vi "Status Display Configuration.vi"(0 "VISA resource name (in)":refnum<visa-resource-name>, 2 "Unit Address (-1)":i32=-1, 5 "error in (no error)":errorcluster, 6 "Retry Attempts (0)":i32 min=0) -> (14 "VISA resource name (out)":refnum<visa-resource-name>, 15 "Decimal Point":T4, 16 "Temperature Units":T3, 17 "Display Color":T2, 18 "Display Brightness":T1, 19 "error out":errorcluster)   [LabVIEW 2020, in "Omega Platinum Series.lvlib"]
doc: "Get the display configuration for the controller."
uses:
  <instrlib>/RxnRover/OmegaPlatinumSeriesDriver/Omega Platinum Series.lvlib
  <instrlib>/RxnRover/OmegaPlatinumSeriesDriver/Public/Type Defs/Display Decimal Point.ctl
  <instrlib>/RxnRover/OmegaPlatinumSeriesDriver/Public/Type Defs/Display Temperature Units.ctl
  <instrlib>/RxnRover/OmegaPlatinumSeriesDriver/Public/Type Defs/Display Color.ctl
  <instrlib>/RxnRover/OmegaPlatinumSeriesDriver/Public/Type Defs/Display Brightness.ctl
panel:
  out "Command":string
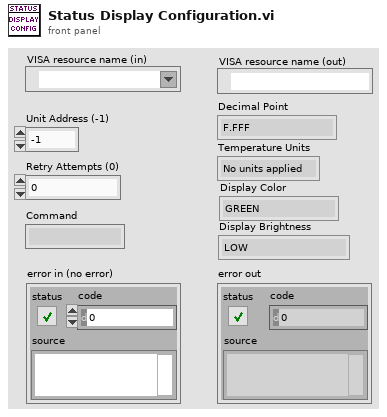
[diagram p1: front panel]
types:
  T1 = typedef "Omega Platinum Series.lvlib/Display Brightness.ctl" = enum16{"LOW", "MEDIUM", "HIGH"}
  T2 = typedef "Omega Platinum Series.lvlib/Display Color.ctl" = enum16{"GREEN", "RED", "AMBER"}
  T3 = typedef "Omega Platinum Series.lvlib/Display Temperature Units.ctl" = enum16{"No units applied", "Celsius", "Fahrenheit"}
  T4 = typedef "Omega Platinum Series.lvlib/Display Decimal Point.ctl" = enum16{"F.FFF", "FF.FF"}
  T5 = typedef "Omega Platinum Series.lvlib/Response.ctl" = cluster{"Unit Address":i32, "Command Class":string, "Command ID":u32, "Parameters":string}
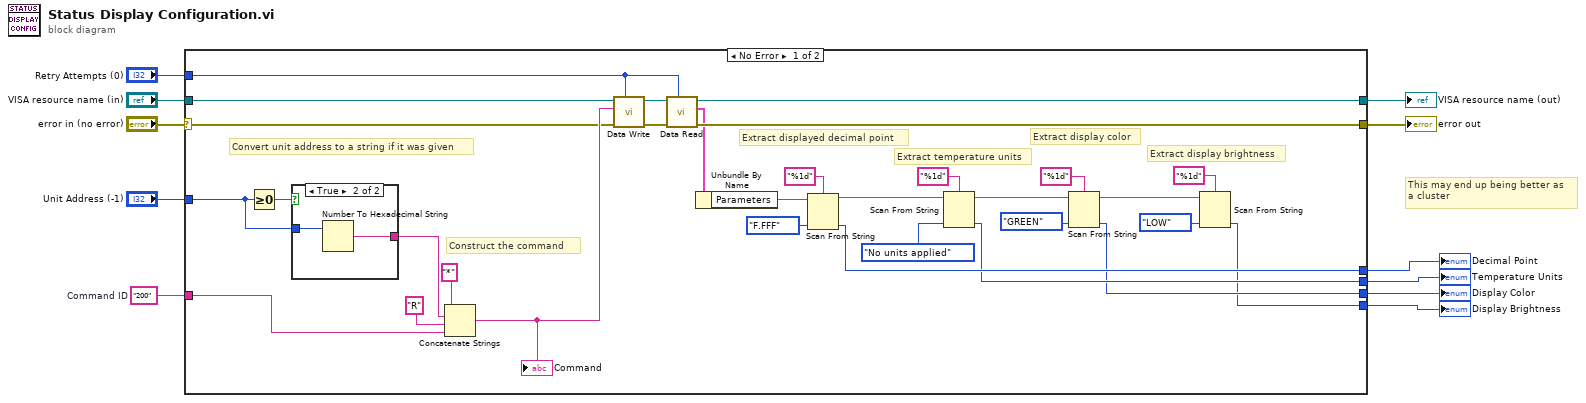
[diagram p0: block diagram]
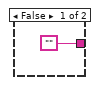
[diagram p2: hidden frame]
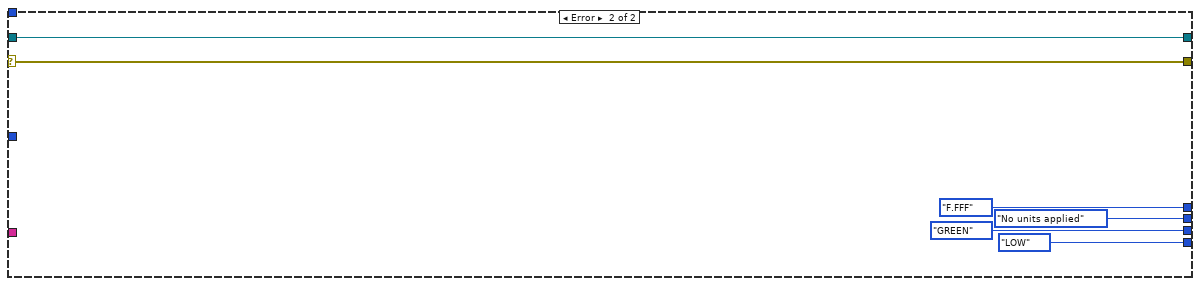
[diagram p3: hidden frame]
diagram:
  w11 = "200"  # Command ID
  # "This may end up being better as\na cluster"
  n1 = case shown="No Error" "error in (no error)" {
    selector: "error in (no error)" -> [w36 w51]
    tunnel: w11 -> [w30 _]
    tunnel: "Unit Address (-1)" -> [w40 _]
    tunnel: [w32 w51] -> w8
    tunnel: "VISA resource name (in)" -> [w38 w50]
    tunnel: [w33 w50] -> w6
    tunnel: [w16 Display_Decimal_Point."F.FFF" ("Decimal Point")] -> w5
    tunnel: [w15 Display_Temperature_Units."No units applied" ("Temperature Units")] -> w4
    tunnel: [w14 Display_Color."GREEN" ("Display Color")] -> w3
    tunnel: [w13 Display_Brightness."LOW" ("Display Brightness")] -> w2
    tunnel: "Retry Attempts (0)" -> [w12 _]
    frame No Error {
      # "Extract display brightness"
      # "Extract display color"
      # "Extract temperature units"
      # "Extract displayed decimal point"
      # "Convert unit address to a string if it was given"
      # "Construct the command"
      n2 = Greater Or Equal To 0?(x=w40) -> (x >= 0?=w42:bool)
      n3 = case shown="True" w42 {
        tunnel: w40 -> [_ w45]
        tunnel: ["" w44] -> w39
        frame False {
        }
        frame True {
          n4 = Number To Hexadecimal String(2:w45) -> (0:w44:string)  [unwired: 1 in]
        }
      }
      n5 = Concatenate Strings("*" ("string"), w39, "R" ("string"), w30) -> (w37:string)
      "Command" <- w37
      n6 = call <instrlib>:"Data Write.vi"("Retry Attempts (0)"=w12, "error in (no error)"=w36, "Command"=w37, "VISA Refnum in"=w38) -> ("error out"=w35:errorcluster, "VISA Refnum out"=w34:refnum<visa-resource-name>)  [unwired: 6 in]
      n7 = call <instrlib>:"Data Read.vi"("Retry Attempts (0)"=w12, "error in (no error)"=w35, "VISA Refnum in"=w34) -> ("error out"=w32:errorcluster, "Response Cluster"=w29:T5, "VISA Refnum out"=w33:refnum<visa-resource-name>)  [unwired: 5 in, 1 out]
      n8 = Unbundle By Name(w29) -> ("Parameters"=w27:string)
      n9 = Scan From String(format string="%1d", input string=w27, default 1=Display_Decimal_Point."F.FFF" ("Decimal Point")) -> (remaining string=w25:string, output 1=w16:T4)  [unwired: 2 in, 2 out]
      n10 = Scan From String(format string="%1d", input string=w25, default 1=Display_Temperature_Units."No units applied" ("Temperature Units")) -> (remaining string=w24:string, output 1=w15:T3)  [unwired: 2 in, 2 out]
      n11 = Scan From String(format string="%1d", input string=w24, default 1=Display_Color."GREEN" ("Display Color")) -> (remaining string=w23:string, output 1=w14:T2)  [unwired: 2 in, 2 out]
      n12 = Scan From String(format string="%1d", input string=w23, default 1=Display_Brightness."LOW" ("Display Brightness")) -> (output 1=w13:T1)  [unwired: 2 in, 3 out]
    }
    frame Error {
    }
  }
  "error out" <- w8
  "VISA resource name (out)" <- w6
  "Decimal Point" <- w5
  "Temperature Units" <- w4
  "Display Color" <- w3
  "Display Brightness" <- w2
